vi "json Insert Variant - string path.vi"(8 "error in (no error)":errorcluster, 9 "anything":variant, 10 "path":string, 11 "JSON Document in":refnum<class "JSON Document.lvclass">) -> (0 "error out":errorcluster, 3 "JSON Document out":refnum<class "JSON Document.lvclass">)   [LabVIEW 2015, in "JSON Document.lvclass"]
uses:
  JSON Document.lvclass
  JSON Document.lvclass/JSON Document.ctl
  rapidjson wrapper/rapidjson wrapper.lvlib
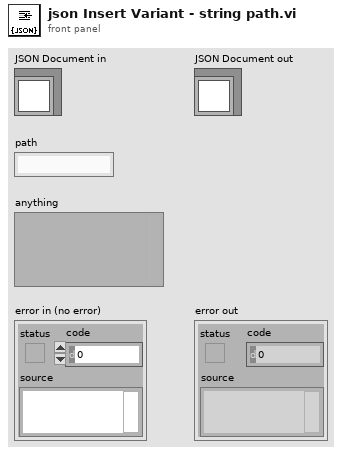
[diagram p1: front panel]
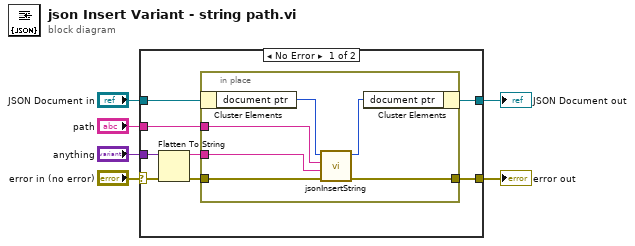
[diagram p0: block diagram]
diagram:
  n1 = case shown="No Error" "error in (no error)" {
    selector: "error in (no error)" -> [w9 w22]
    tunnel: [w11 w22] -> w5
    tunnel: [w13 w21] -> w3
    tunnel: "JSON Document in" -> [w14 w21]
    tunnel: "anything" -> [w10 _]
    tunnel: "path" -> [w12 _]
    frame No Error {
      n2 = Flatten To String(anything=w10, error in (no error)=w9) -> (data string=w7:string, error out=w8:errorcluster)  [unwired: 2 in, 1 out]
      n3 = in-place {
        in-place-border: w12 -> [w18]
        in-place-border: w8 -> [w17]
        in-place-border: [w16] -> w11
        in-place-border: w7 -> [w15]
        n4 = in-place-cluster #1(w14) -> ("document ptr"=w20:i64)
        n5 = call "jsonInsertString.vi"("error in (no error)"=w17, "value"=w15, "path"=w18, "d in"=w20) -> ("error out"=w16:errorcluster, "d out"=w19:i64)  [unwired: 6 in]
        n6 = in-place-cluster #1("document ptr"=w19) -> (w13:refnum<class "JSON Document.lvclass">)
      }
    }
    frame Error {
    }
  }
  "error out" <- w5
  "JSON Document out" <- w3
